vi "Flash Stop Live Mode.vi"(8 "error in (no error)":errorcluster, 11 "Orca-Flash 4.0 V2 in":refnum<class "Orca-Flash 4.0 V2.lvclass">) -> (0 "error out":errorcluster, 3 "Orca-Flash 4.0 V2 out":refnum<class "Orca-Flash 4.0 V2.lvclass">)   [LabVIEW 2018, in "Orca-Flash 4.0 V2.lvlib" / "Orca-Flash 4.0 V2.lvclass"]
uses:
  Orca-Flash 4.0 V2.lvclass
  C:/LVCUR/flash-gordon/Hardware/Camera/Camera.lvclass
  Orca-Flash 4.0 V2.lvclass/Orca-Flash 4.0 V2.ctl
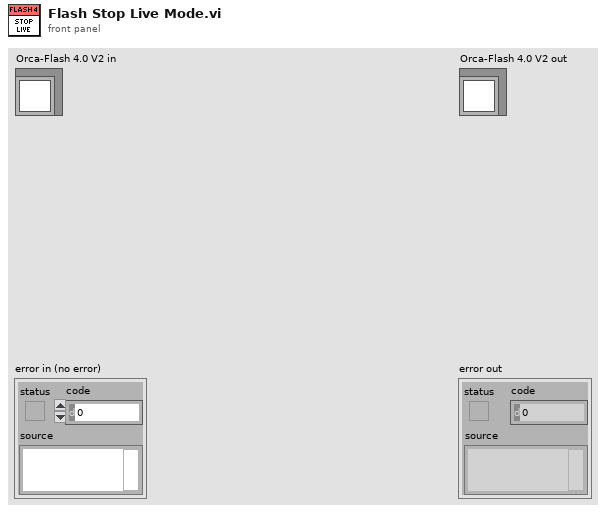
[diagram p1: front panel]
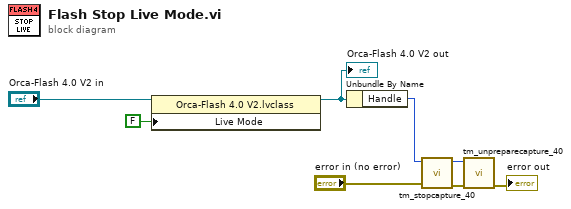
[diagram p0: block diagram]
diagram:
  n1 = property class="Orca-Flash 4.0 V2.lvclass"(reference="Orca-Flash 4.0 V2 in", "Live Mode"=FALSE) -> (reference out=w6:refnum<class "Orca-Flash 4.0 V2.lvclass">)  [unwired: 1 in, 1 out]
  "Orca-Flash 4.0 V2 out" <- w6
  n2 = Unbundle By Name(w6) -> ("Handle"=w3:u32)
  n3 = call <userlib>:"tm_stopcapture_40.vi"("error in (no error)"="error in (no error)", "Handle in"=w3) -> ("error out"=w5:errorcluster, "Handle out"=w4:u32)  [unwired: 8 in]
  n4 = call <userlib>:"tm_unpreparecapture_40.vi"("error in (no error)"=w5, "Handle in"=w4) -> ("error out"=→"error out":errorcluster)  [unwired: 8 in, 1 out]
